vi "Process Counter Signals.vi"(8 "Values Received":dbl[](array[numeric]), 9 "Prot Ctr Values In":dbl[](array[numeric]), 10 "Invalid Counts In":dbl[](array[numeric]), 11 "Frame Settings In":T1 {"Protection Configurations"."CRC Channels"."Data Type" items=["Signed", "Unsigned", "IEEE Float"]}) -> (1 "Prot Ctr Values Out":dbl[](array[numeric]), 2 "Invalid Counts Out":dbl[](array[numeric]), 3 "Frame Settings Out":T1 {"Protection Configurations"."CRC Channels"."Data Type" items=["Signed", "Unsigned", "IEEE Float"]})   [LabVIEW 2019, in "Protection and Counter Addon Engine.lvlib"]
uses:
  Protection and Counter Addon Engine.lvlib
  SubModules/Frame-Protection-Support/Source/Shared/Types/RT Exported Signal Settings.ctl
  SubModules/Frame-Protection-Support/Source/Shared/Types/Exported Counter Settings.ctl
  SubModules/Frame-Protection-Support/Source/Engine/Types/RT Protection Configuration.ctl
  SubModules/Frame-Protection-Support/Source/Shared/Types/Protection Type.ctl
  SubModules/Frame-Protection-Support/Source/Shared/Types/XNET Signal Configuration.ctl
  SubModules/Frame-Protection-Support/Source/Engine/Types/RT Frame Settings.ctl
  SubModules/Frame-Protection-Support/Source/Shared/Types/Exported Frame Type.ctl
  SubModules/Frame-Protection-Support/Source/Shared/Types/Exported Event Trigger Type.ctl
  <vilib>/NI VeriStand/Custom Device Tools/Custom Device Utility Library/Custom Device Utility Library.lvlib
  SubModules/Frame-Protection-Support/Source/Shared/Protection and Counter Support Shared.lvlib
  SubModules/Frame-Protection-Support/Source/Engine/Protection and Counter Support Engine.lvlib
panel:
  out "Signal Settings Out":T8 {"Protection Configuration"."CRC Channels"."Data Type" items=["Signed", "Unsigned", "IEEE Float"]}
  in  "Signal Settings In":T8 {"Protection Configuration"."CRC Channels"."Data Type" items=["Signed", "Unsigned", "IEEE Float"]}
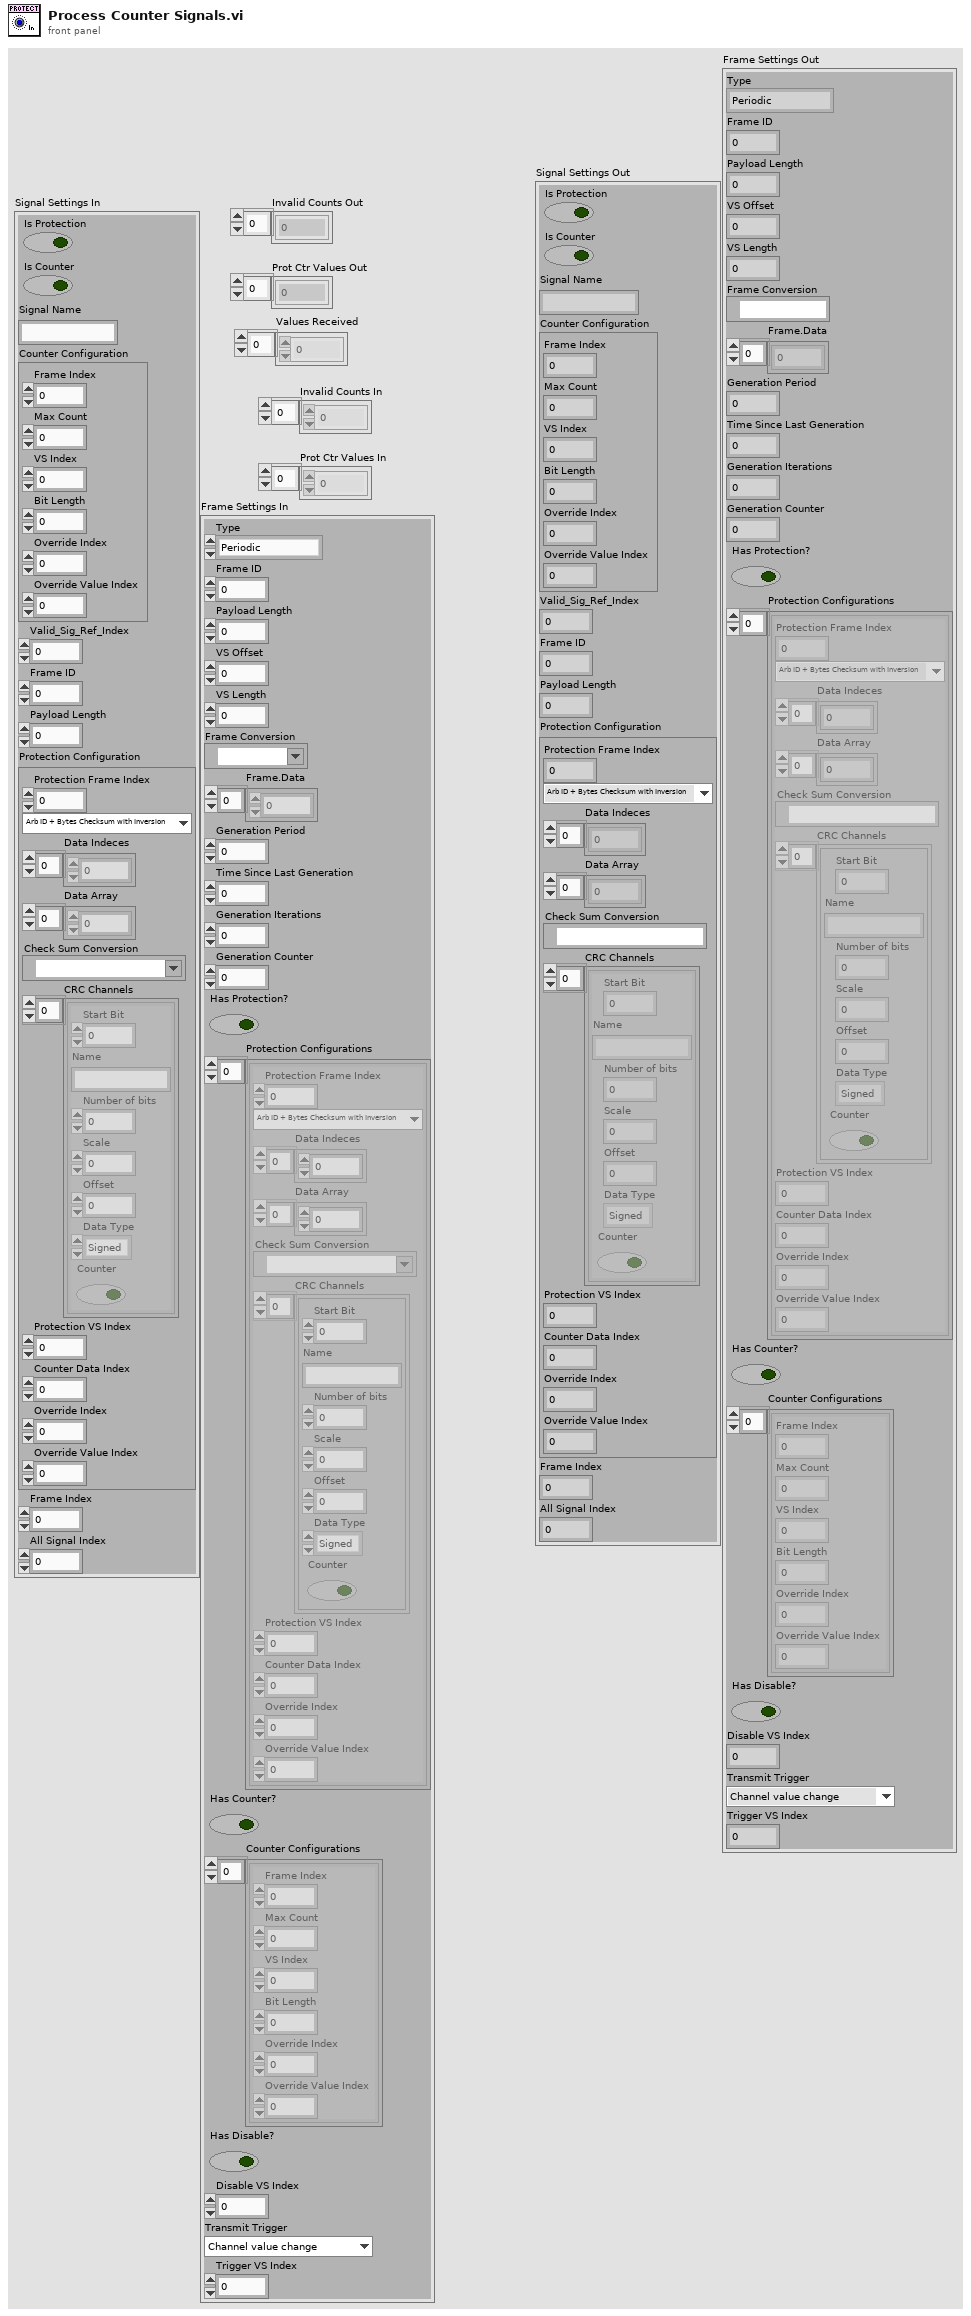
[diagram p1: front panel]
types:
  T1 = typedef "Protection and Counter Support Engine.lvlib/RT Frame Settings.ctl" = cluster{"Type":T2, "Frame ID":u32, "Payload Length":u32, "VS Offset":i32, "VS Length":i32, "Frame Conversion":refnum<k21>, "Frame.Data":dbl[], "Generation Period":u32, "Time Since Last Generation":u32, "Generation Iterations":u32, "Generation Counter":u32, "Has Protection?":bool, "Protection Configurations":T3[], "Has Counter?":bool, "Counter Configurations":T6[], "Has Disable?":bool, "Disable VS Index":i32, "Transmit Trigger":T7, "Trigger VS Index":i32}
  T2 = typedef "Protection and Counter Support Shared.lvlib/Exported Frame Type.ctl" = enum16{"Periodic", "Event", "Periodic/Event"}
  T3 = typedef "Protection and Counter Support Engine.lvlib/RT Protection Configuration.ctl" = cluster{"Protection Frame Index":i32, "Protection Type":T4, "Data Indeces":i32[], "Data Array":dbl[], "Check Sum Conversion":refnum<k21>, "CRC Channels":T5[], "Protection VS Index":i32, "Counter Data Index":i32, "Override Index":i32, "Override Value Index":i32}
  T4 = typedef "Protection and Counter Support Shared.lvlib/Protection Type.ctl" = enum16{"Arb ID + Bytes Checksum with Inversion", "Arb ID + Bytes CRC with Inversion", "Reversed Raw Signal Checksum with Inversion", "Concatenated Two's Compliment"}
  T5 = typedef "Protection and Counter Support Shared.lvlib/XNET Signal Configuration.ctl" = cluster{"Start Bit":i32, "Name":string, "Number of bits":i32, "Scale":dbl, "Offset":dbl, "Data Type":u32, "Counter":bool}
  T6 = typedef "Protection and Counter Support Shared.lvlib/Exported Counter Settings.ctl" = cluster{"Frame Index":i32, "Max Count":dbl, "VS Index":i32, "Bit Length":i64, "Override Index":i32, "Override Value Index":i32}
  T7 = typedef "Protection and Counter Support Shared.lvlib/Exported Event Trigger Type.ctl" = enum16{"Channel value change", "Trigger channel (not zero)", "Channel value change or trigger channel (not zero)", "Trigger channel (any value change)", "Channel value change or trigger channel (any value change)"}
  T8 = typedef "RT Exported Signal Settings.ctl" = cluster{"Is Protection":bool, "Is Counter":bool, "Signal Name":string, "Counter Configuration":T6, "Valid_Sig_Ref_Index":i32, "Frame ID":u32, "Payload Length":u32, "Protection Configuration":T3, "Frame Index":i32, "All Signal Index":i32}
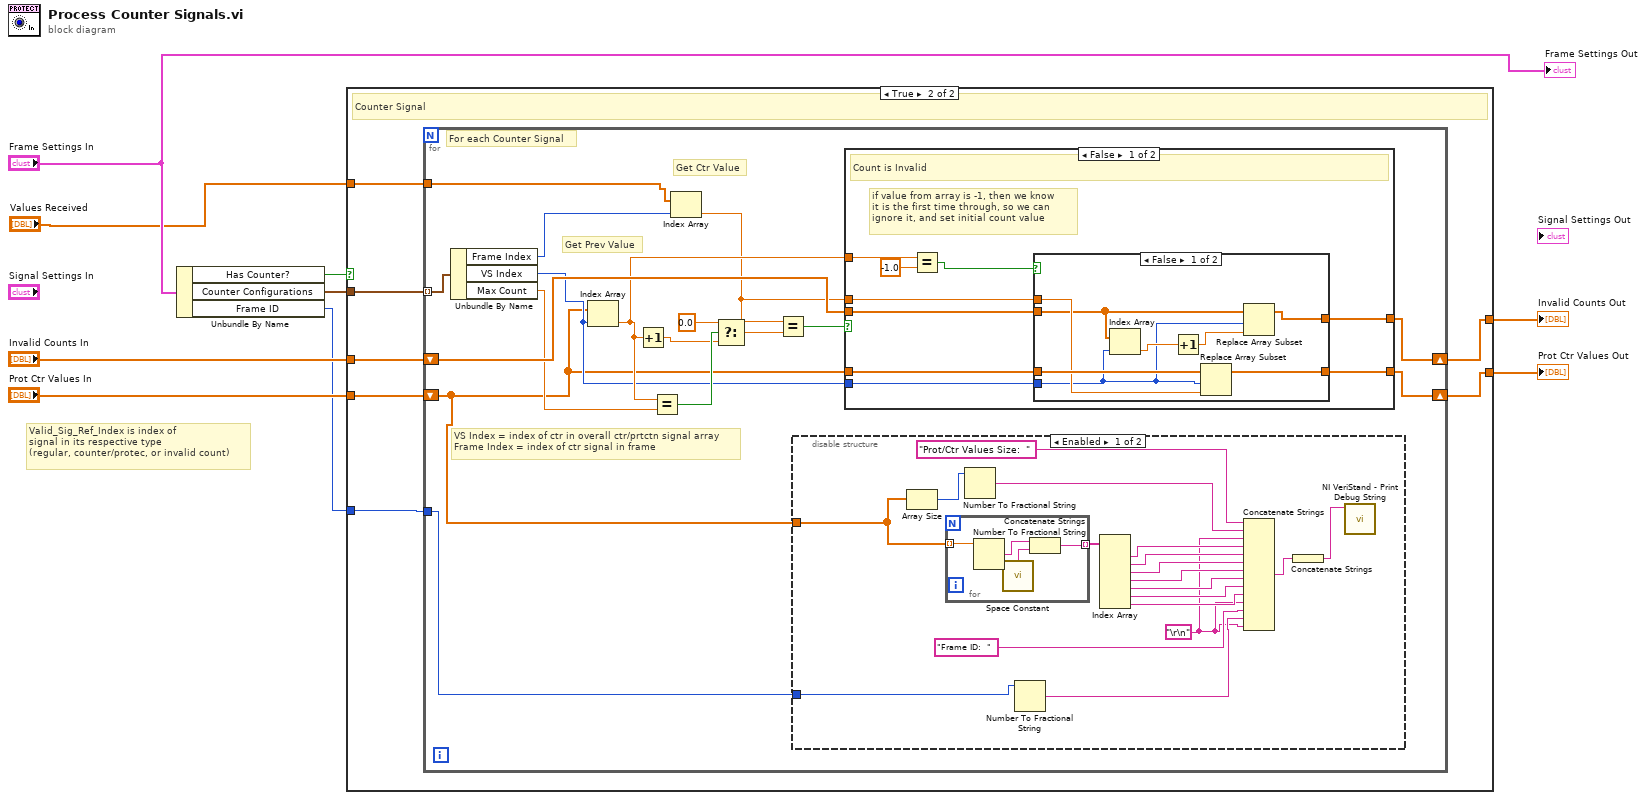
[diagram p0: block diagram]
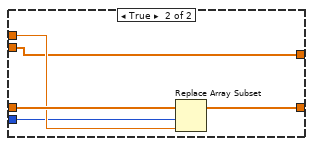
[diagram p4: hidden frame]
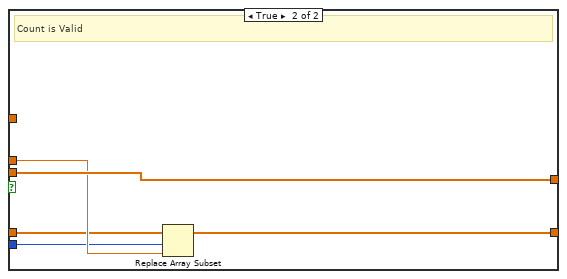
[diagram p5: hidden frame]
diagram:
  # "Valid_Sig_Ref_Index is index of \nsignal in its respective type \n(regular, counter/protec, or invalid count)"
  n1 = Unbundle By Name("Frame Settings In") -> ("Has Counter?"=w3:bool, "Counter Configurations"=w9:T6[], "Frame ID"=w1:u32)
  n2 = case shown="True" w3 {
    tunnel: "Values Received" -> [_ w15]
    tunnel: "Invalid Counts In" -> [w11 w14]
    tunnel: w9 -> [_ w13]
    tunnel: [w11 w18] -> w6
    tunnel: "Prot Ctr Values In" -> [w10 w16]
    tunnel: [w10 w17] -> w8
    tunnel: w1 -> [_ w12]
    frame False {
    }
    frame True {
      # "Counter Signal"
      n3 = for {
        tunnel: w15 -> [w23]
        tunnel: w13 -> [w26] mode=indexing
        shift-right: [w35] -> w18
        shift-left: w14 -> [w28]
        shift-right: [w34] -> w17
        shift-left: w16 -> [w19]
        tunnel: w12 -> [w20]
        # "Get Ctr Value"
        # "For each Counter Signal"
        # "VS Index = index of ctr in overall ctr/prtctn signal array\nFrame Index = index of ctr signal in frame"
        # "Get Prev Value"
        n4 = Unbundle By Name(w26) -> ("Frame Index"=w22:i32, "VS Index"=w24:i32, "Max Count"=w25:dbl)
        n5 = Index Array(array=w19, index=w24) -> (element=w27:dbl)
        n6 = Increment(x=w27) -> (x+1=w31:dbl)
        n7 = Equal?(x=w27, y=w25) -> (x = y?=w33:bool)
        n8 = Index Array(array=w23, index=w22) -> (element=w21:dbl)
        n9 = Select(t=0.0, s=w33, f=w31) -> (s? t:f=w30:dbl)
        n10 = Equal?(x=w21, y=w30) -> (x = y?=w29:bool)
        n11 = disable-structure shown="Enabled" {
          disable-tunnel: w19 -> [w41 _]
          disable-tunnel: w20 -> [w38 _]
          frame Enabled {
            w36 = "\r\n"
            n12 = Array Size(array=w41) -> (size(s)=w53:i32)
            n13 = for {
              tunnel: w41 -> [w55] mode=indexing
              tunnel: [w54] -> w50 mode=indexing
              n14 = Number To Fractional String(number=w55) -> (F-format string=w57:string)  [unwired: 3 in]
              n15 = call <vilib>:"Space Constant.vi"() -> ("String"=w56:string)
              n16 = Concatenate Strings(w57, w56) -> (w54:string)
            }
            n17 = Number To Fractional String(number=w53) -> (F-format string=w51:string)  [unwired: 3 in]
            n18 = Number To Fractional String(number=w38) -> (F-format string=w37:string)  [unwired: 3 in]
            n19 = Index Array(array=w50) -> (element #1=w49:string, element #2=w48:string, element #3=w47:string, element #4=w46:string, element #5=w45:string, element #6=w44:string, element #7=w40:string)  [unwired: 7 in]
            n20 = Concatenate Strings("Prot/Ctr Values Size:  ", w51, w36, w49, w48, w47, w46, w45, w44, w40, w36, "Frame ID:  ", w37, w36) -> (w43:string)
            n21 = Concatenate Strings(w43) -> (w42:string)
            n22 = call <vilib>:"NI VeriStand - Print Debug String.vi"("Message"=w42) -> ()  [unwired: 10 in, 1 out]
          }
          frame Disabled {
          }
        }
        n23 = case shown="False" w29 {
          tunnel: w28 -> [w63 w84]
          tunnel: [w62 w84] -> w35
          tunnel: w21 -> [w65 w83]
          tunnel: [w64 w82] -> w34
          tunnel: w19 -> [w66 w81]
          tunnel: w27 -> [w61 _]
          tunnel: w24 -> [w58 w80]
          frame False {
            # "if value from array is -1, then we know \nit is the first time through, so we can\nignore it, and set initial count value"
            # "Count is Invalid"
            n24 = Equal?(x=w61, y=-1.0) -> (x = y?=w59:bool)
            n25 = case shown="False" w59 {
              tunnel: w66 -> [w74 w79]
              tunnel: w65 -> [w73 w78]
              tunnel: [w72 w77] -> w64
              tunnel: w63 -> [w71 w76]
              tunnel: [w68 w76] -> w62
              tunnel: w58 -> [w67 w75]
              frame False {
                n26 = Index Array(array=w71, index=w67) -> (element=w70:dbl)
                n27 = Increment(x=w70) -> (x+1=w69:dbl)
                n28 = Replace Array Subset(array=w74, new element=w73, index=w67) -> (w72:dbl[])
                n29 = Replace Array Subset(array=w71, new element=w69, index=w67) -> (w68:dbl[])
              }
              frame True {
                n30 = Replace Array Subset(array=w79, new element=w78, index=w75) -> (w77:dbl[])
              }
            }
          }
          frame True {
            # "Count is Valid"
            n31 = Replace Array Subset(array=w81, new element=w83, index=w80) -> (w82:dbl[])
          }
        }
      }
    }
  }
  "Prot Ctr Values Out" <- w8
  "Invalid Counts Out" <- w6
  "Frame Settings Out" <- "Frame Settings In"
